vi "trend.vi"(2 "jumpBool":bool, 3 "AD":dbl, 4 "runMin":dbl, 5 "Compensate1":dbl) -> (0 "Compensate1Out":dbl, 1 "changeSymbol":dbl)   [LabVIEW 2018]
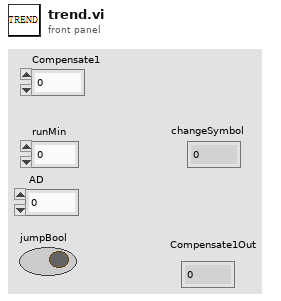
[diagram p1: front panel]
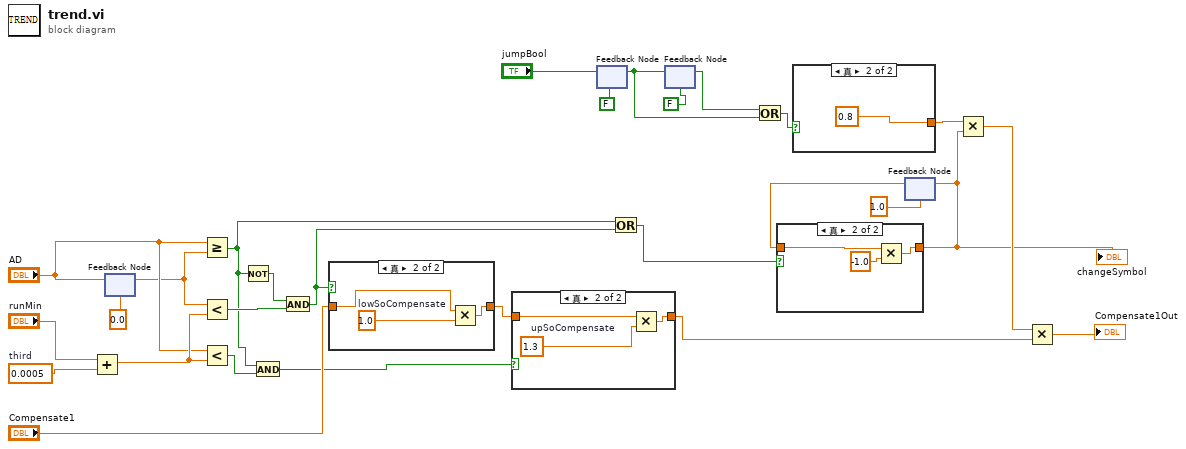
[diagram p0: block diagram]
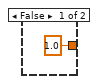
[diagram p2: hidden frame]
diagram:
  w26 = 0.0005  # third
  n1 = Add(x="runMin", y=w26) -> (x+y=w24:dbl)
  n2 = feedback #1(0.0) -> (w22:dbl)
  n3 = feedback-in #1("AD") -> ()
  n4 = Greater Or Equal?(x="AD", y=w22) -> (x >= y?=w16:bool)
  n5 = Less?(x=w22, y=w24) -> (x < y?=w20:bool)
  n6 = Less?(x="AD", y=w24) -> (x < y?=w17:bool)
  n7 = Not(x=w16) -> (.not. x?=w21:bool)
  n8 = And(x=w16, y=w17) -> (x .and. y?=w15:bool)
  n9 = And(x=w21, y=w20) -> (x .and. y?=w19:bool)
  n10 = case shown="真" w19 {
    tunnel: "Compensate1" -> [w29 w32]
    tunnel: [w29 w30] -> w18
    frame False {
    }
    frame True {
      w31 = 1.0  # lowSoCompensate
      n11 = Multiply(x=w32, y=w31) -> (x*y=w30:dbl)
    }
  }
  n12 = case shown="真" w15 {
    tunnel: w18 -> [w33 w36]
    tunnel: [w33 w34] -> w5
    frame False {
    }
    frame True {
      w35 = 1.3  # upSoCompensate
      n13 = Multiply(x=w36, y=w35) -> (x*y=w34:dbl)
    }
  }
  n14 = feedback #2(FALSE) -> (w6:bool)
  n15 = feedback-in #2("jumpBool") -> ()
  n16 = Or(x=w16, y=w19) -> (x .or. y?=w8:bool)
  n17 = feedback #3(FALSE) -> (w7:bool)
  n18 = feedback-in #3(w6) -> ()
  n19 = Or(x=w7, y=w6) -> (x .or. y?=w10:bool)
  n20 = case shown="真" w10 {
    tunnel: [1.0 0.8] -> w2
    frame False {
    }
    frame True {
    }
  }
  n21 = feedback #4(1.0) -> (w14:dbl)
  n22 = case shown="真" w8 {
    tunnel: [w39 w40] -> w1
    tunnel: w14 -> [w39 w41]
    frame False {
    }
    frame True {
      n23 = Multiply(x=w41, y=-1.0) -> (x*y=w40:dbl)
    }
  }
  "changeSymbol" <- w1
  n24 = feedback-in #4(w1) -> ()
  n25 = Multiply(x=w2, y=w1) -> (x*y=w3:dbl)
  n26 = Multiply(x=w3, y=w5) -> (x*y=→"Compensate1Out":dbl)
